vi "S2DS_GR-test.vi"(9 "Write command":string, 10 "format string":string, 11 "VISA Refnum in":refnum<visa-resource-name>) -> (0 "Error in parsing the value":errorcluster, 2 "GR Value":dbl, 3 "VISA Refnum out":refnum<visa-resource-name>)   [LabVIEW 2025]
panel:
  out "error in response \nfrom instrument":errorcluster
  out "read buffer":string
  # "Test command based reading from instrument..."
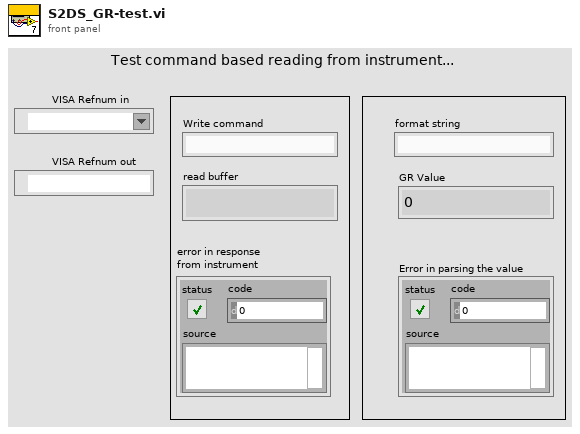
[diagram p1: front panel]
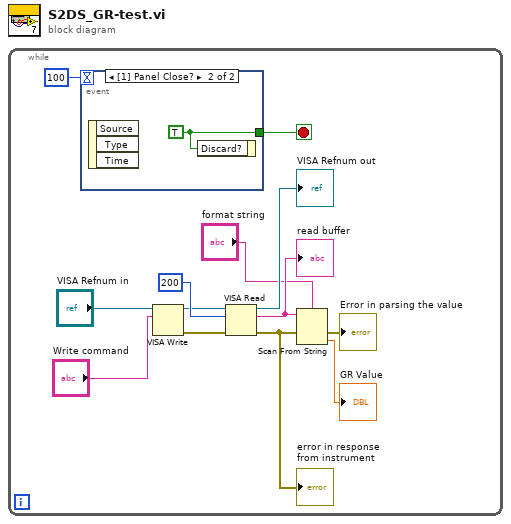
[diagram p0: block diagram]
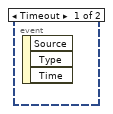
[diagram p2: hidden frame]
diagram:
  n1 = while {
    stop <- w1 stop-if-true
    n2 = event shown="[1] Panel Close?" {
      selector: _ -> [_ _]
      dyn-events: _ -> [_ _]
      timeout: 100 -> [_ _]
      tunnel: [_ w14] -> w1
      event Timeout {
        n3 = event-data() -> ()  [unwired: 1 in, 3 out]
      }
      event Panel Close? {
        w14 = TRUE ("Discard?")
        n4 = event-data() -> ()  [unwired: 1 in, 3 out]
        n5 = event-data("Discard?"=w14) -> ()  [unwired: 1 in, 1 out]
      }
    }
    n6 = VISA Write(VISA resource name="VISA Refnum in", write buffer="Write command") -> (VISA resource name out=w5:refnum<visa-resource-name>, error out=w4:errorcluster)  [unwired: 1 in, 1 out]
    n7 = VISA Read(VISA resource name=w5, byte count=u32 200, error in (no error)=w4) -> (VISA resource name out=→"VISA Refnum out":refnum<visa-resource-name>, read buffer=w7:string, error out=w6:errorcluster)  [unwired: 1 out]
    "read buffer" <- w7
    "error in response \nfrom instrument" <- w6
    n8 = Scan From String(format string="format string", input string=w7, error in=w6) -> (error out=→"Error in parsing the value":errorcluster, output 1=→"GR Value":dbl)  [unwired: 2 in, 2 out]
  }
